vi "Pack for gRPC.vi"(8 "error in":errorcluster, 9 "configuration / results":enum16{"Configuration", "Results"}(ring), 10 "data value":variant, 11 "measurement plugin in":refnum<class "FPT NoiseFigure.lvclass">) -> (0 "error out":errorcluster, 2 "any":T1, 3 "measurement plugin out":refnum<class "FPT NoiseFigure.lvclass">)   [LabVIEW 2023, in "FPT NoiseFigure.lvclass"]
uses:
  FPT NoiseFigure.lvclass
  <vilib>/gRPC/LabVIEW gRPC Library/Shared/Any.ctl
  Measurement Configuration.ctl
  Measurement Results.ctl
  2eca732d-dbaa-43bf-a7dd-ede2da65bc1b.vi
  a6012965-5700-4384-8228-972e71b6560c.vi
  <vilib>/gRPC/LabVIEW gRPC Library/Server API/Translate Protobuf Error.vi
  <vilib>/AdvancedString/1D String Array to Delimited String.vi
  <vilib>/gRPC/LabVIEW gRPC Library/Server API/Server/Get Server DLL Path.vi
  FPT NoiseFigure.lvclass/FPT NoiseFigure.ctl
  <vilib>/Plug-In SDKs/Measurements/Measurement Plugin Service/Measurement Plugin Service.lvclass
  <vilib>/gRPC/LabVIEW gRPC Library/grpc-lvsupport-release.lvlib
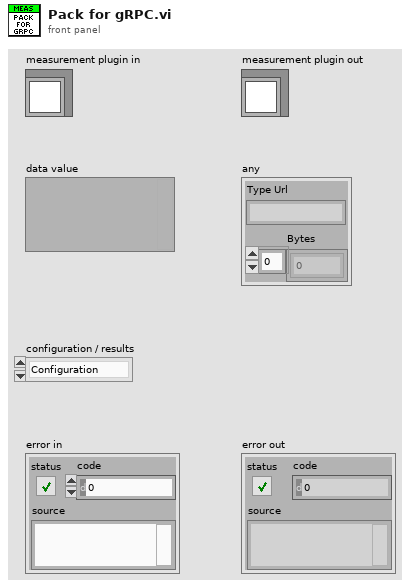
[diagram p1: front panel]
types:
  T1 = typedef "grpc-lvsupport-release.lvlib/Any.ctl" = cluster{"Type Url":string, "Bytes":u8[]}
  T2 = typedef "grpc-lvsupport-release.lvlib/grpcId.ctl" = u64
  T3 = typedef "FPT NoiseFigure.lvclass/Measurement Configuration.ctl" = cluster{"Automation Test":bool, "Power sequencing file path":string, "RFmx name":string, "RFmx port":string, "DUT Max Gain (dB)":dbl, "DUT Max Noise Figure (dB)":dbl, "Reference Level Mode":enum32{"Manual", "Recommend"}, "Reference Level (dBm)":dbl, "Preamp Enabled":i32, "RFmx attenuation mode":enum32{"<None>", "Constant Attenuation", "s2p File"}, "RFmx external attenuation (dB)":dbl, "RFmx s-parameters orientation":enum32{"Port1 Towards DUT", "Port2 Towards DUT"}, "RFmx s2p file path":string, "Switch Name":string, "Switch Connection":string, "ENS SMU Name":string, "ENS SMU Channel":string, "Action":u32, "Measurement Bandwidth (Hz)":dbl, "Measurement Interval (s)":dbl, "NF Cal Setup ID":string, "DUT Type":i32, "Frequency List Mode":enum32{"Step", "Points", "Frequency List"}, "Step - Start Frequency ":dbl, "Step - Stop Frequency":dbl, "Step - Step Size":dbl, "Points - Start Frequency":dbl, "Points - Stop Frequency":dbl, "Points - Number of Points":i32, "FreqList - Frequency List":dbl[], "Averaging Enabled":bool, "Averaging Count":i32, "Noise Source Type":i32, "Noise Source RFSG Port":string, "Noise Source Cold Temperature (K)":dbl, "Noise Source Off Temperature (K)":dbl, "ENR Freq (Hz)":dbl[], "ENR (dB)":dbl[], "DUT Input_Compensation Enabled":bool, "DUT Input_Temperation (K)":dbl, "DUT Input_Loss Freq (Hz)":dbl[], "DUT Input_Loss (dB)":dbl[], "DUT Output_Compensation Enabled":bool, "DUT Output_Temperation (K)":dbl, "DUT Output_Loss Freq (Hz)":dbl[], "DUT Output_Loss (dB)":dbl[], "Calibration_Compensation Enabled":bool, "Calibration_Temperation (K)":dbl, "Calibration_Loss Freq (Hz)":dbl[], "Calibration_Loss (dB)":dbl[], "Noise Source_Compensation Enabled":bool, "Noise Source_Temperation (K)":dbl, "Noise Source_Loss Freq (Hz)":dbl[], "Noise Source_Loss (dB)":dbl[], "DUT Input Loss S2P File Path":string, "DUT Input Loss S-Parameter Orientation":i32, "DUT Output Loss S2P File Path":string, "DUT Output Loss S-Parameter Orientation":i32, "Calibration Loss S2P File Path":string, "Calibration Loss S-Parameter Orientation":i32, "Noise Source Loss S2P File Path":string, "Noise Source Loss S-Parameter Orientation":i32, "Power sequencing file validity check":bool}
  T4 = typedef "FPT NoiseFigure.lvclass/Measurement Results.ctl" = cluster{"Status":string, "DUT NF vs Freq":dbl[][], "Analyzer NF vs Freq":dbl[][], "DUT NF (mean)":dbl, "Analyzer NF (mean)":dbl}
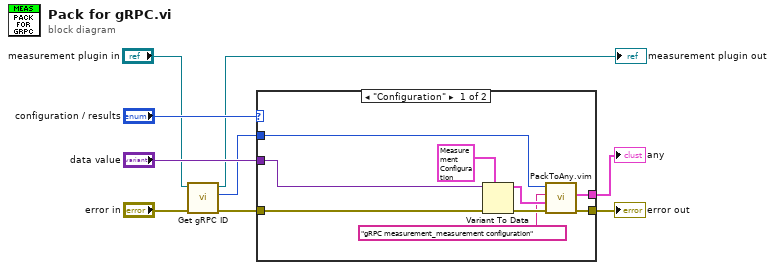
[diagram p0: block diagram]
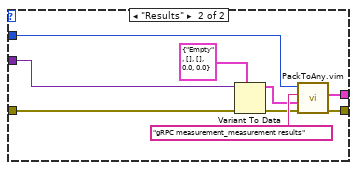
[diagram p2: hidden frame]
diagram:
  n1 = call <vilib>:"Get gRPC ID.vi"("error in"="error in", "measurement plugin service in"="measurement plugin in") -> ("error out"=w4:errorcluster, "gRPC ID"=w1:T2, "measurement plugin service out"=→"measurement plugin out":refnum<class "FPT NoiseFigure.lvclass">)  [unwired: 7 in]
  n2 = case shown="\"Configuration\"" "configuration / results" {
    tunnel: w4 -> [w18 w27]
    tunnel: "data value" -> [w17 w26]
    tunnel: w1 -> [w14 w22]
    tunnel: [w16 w24] -> w8
    tunnel: [w15 w23] -> w7
    frame "Configuration" {
      n3 = Variant To Data(error in=w18, type=T3 {"Automation Test"=FALSE, "Power sequencing file path"="Lorem ipsum dolor sit", "RFmx name"="5842_0", "RFmx port"="Lorem ipsum dolor sit", "DUT Max Gain (dB)"=3.0, "DUT Max Noise Figure (dB)"=1.2, "Reference Level Mode"=enum."Manual", "Reference Level (dBm)"=1.2, "Preamp Enabled"=0, "RFmx attenuation mode"=enum."Constant Attenuation", "RFmx external attenuation (dB)"=1.0, "RFmx s-parameters orientation"=enum."Port2 Towards DUT", "RFmx s2p file path"="", "Switch Name"="2599_S8", "Switch Connection"="no0->com0", "ENS SMU Name"="", "ENS SMU Channel"="", "Action"=0, "Measurement Bandwidth (Hz)"=4000000.0, "Measurement Interval (s)"=0.1, "NF Cal Setup ID"="SNS_PS_6dB_ENR15_26.5GHz_VI", "DUT Type"=0, "Frequency List Mode"=enum."Step", "Step - Start Frequency "=1000000000.0, "Step - Stop Frequency"=2000000000.0, "Step - Step Size"=100000000.0, "Points - Start Frequency"=1000000000.0, "Points - Stop Frequency"=2000000000.0, "Points - Number of Points"=11, "FreqList - Frequency List"=[4000000000.0, 5000000000.0, 6000000000.0, 7000000000.0, 8000000000.0, 9000000000.0, 10000000000.0, 11000000000.0, 12000000000.0, 13000000000.0, 14000000000.0, 15000000000.0, 16000000000.0, 17000000000.0, 18000000000.0, 19000000000.0, 20000000000.0], "Averaging Enabled"=FALSE, "Averaging Count"=10, "Noise Source Type"=1, "Noise Source RFSG Port"="port1", "Noise Source Cold Temperature (K)"=302.8, "Noise Source Off Temperature (K)"=297.0, "ENR Freq (Hz)"=[6500000000.0], "ENR (dB)"=[15.0], "DUT Input_Compensation Enabled"=FALSE, "DUT Input_Temperation (K)"=297.0, "DUT Input_Loss Freq (Hz)"=array[589 elements], "DUT Input_Loss (dB)"=array[589 elements], "DUT Output_Compensation Enabled"=FALSE, "DUT Output_Temperation (K)"=297.0, "DUT Output_Loss Freq (Hz)"=array[589 elements], "DUT Output_Loss (dB)"=array[589 elements], "Calibration_Compensation Enabled"=FALSE, "Calibration_Temperation (K)"=297.0, "Calibration_Loss Freq (Hz)"=array[589 elements], "Calibration_Loss (dB)"=array[589 elements], "Noise Source_Compensation Enabled"=FALSE, "Noise Source_Temperation (K)"=297.0, "Noise Source_Loss Freq (Hz)"=[], "Noise Source_Loss (dB)"=[], "DUT Input Loss S2P File Path"="", "DUT Input Loss S-Parameter Orientation"=0, "DUT Output Loss S2P File Path"="", "DUT Output Loss S-Parameter Orientation"=0, "Calibration Loss S2P File Path"="", "Calibration Loss S-Parameter Orientation"=0, "Noise Source Loss S2P File Path"="", "Noise Source Loss S-Parameter Orientation"=0, "Power sequencing file validity check"=TRUE} ("measurement configuration"), Variant=w17) -> (data=w13:T3, error out=w12:errorcluster)
      n4 = call "PackToAny.vim"("error in"=w12, "Data To Pack"=w13, "Message Type"="gRPC measurement_measurement configuration", "gRPCid in"=w14) -> ("error out"=w16:errorcluster, "Any"=w15:T1)  [unwired: 5 in, 1 out]
    }
    frame "Results" {
      n5 = Variant To Data(error in=w27, type=T4 {"Status"="Empty", "DUT NF vs Freq"=[], "Analyzer NF vs Freq"=[], "DUT NF (mean)"=0.0, "Analyzer NF (mean)"=0.0} ("Measurement Results"), Variant=w26) -> (data=w20:T4, error out=w19:errorcluster)
      n6 = call "PackToAny.vim"("error in"=w19, "Data To Pack"=w20, "Message Type"="gRPC measurement_measurement results", "gRPCid in"=w22) -> ("error out"=w24:errorcluster, "Any"=w23:T1)  [unwired: 5 in, 1 out]
    }
  }
  "error out" <- w8
  "any" <- w7
